vi "LlenarTabla.vi"(8 "error in (no error)":errorcluster, 11 "Prueba32 in":refnum<class "Prueba03.lvclass">) -> (0 "error out":errorcluster, 3 "Prueba32 out":refnum<class "Prueba03.lvclass">)   [LabVIEW 2019, in "Prueba03.lvclass"]
uses:
  Prueba03.lvclass
  Prueba03.lvclass/Prueba03.ctl
panel:
  out "Tabla_Ext":string[][](table)=[["63"], ["125"], ["250"], ["500"], ["1000"], ["2000"], ["4000"], ["8000"]]
  out "Tabla_Int":string[][](table)
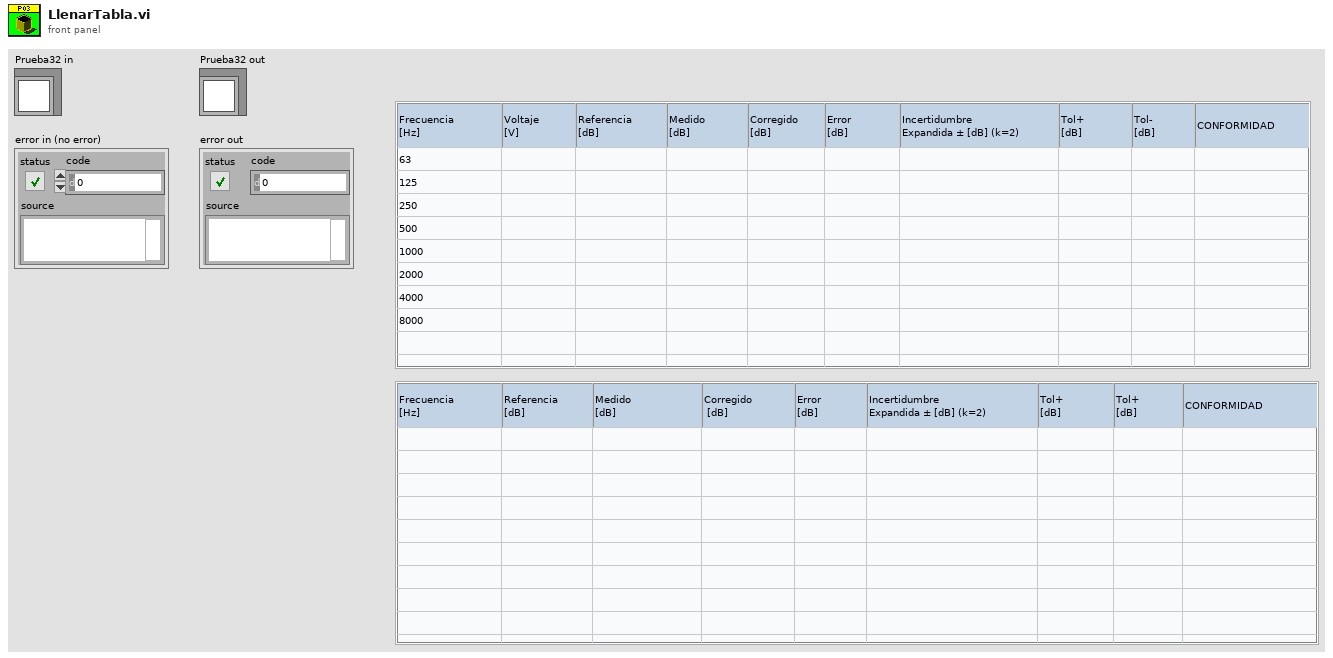
[diagram p1: front panel]
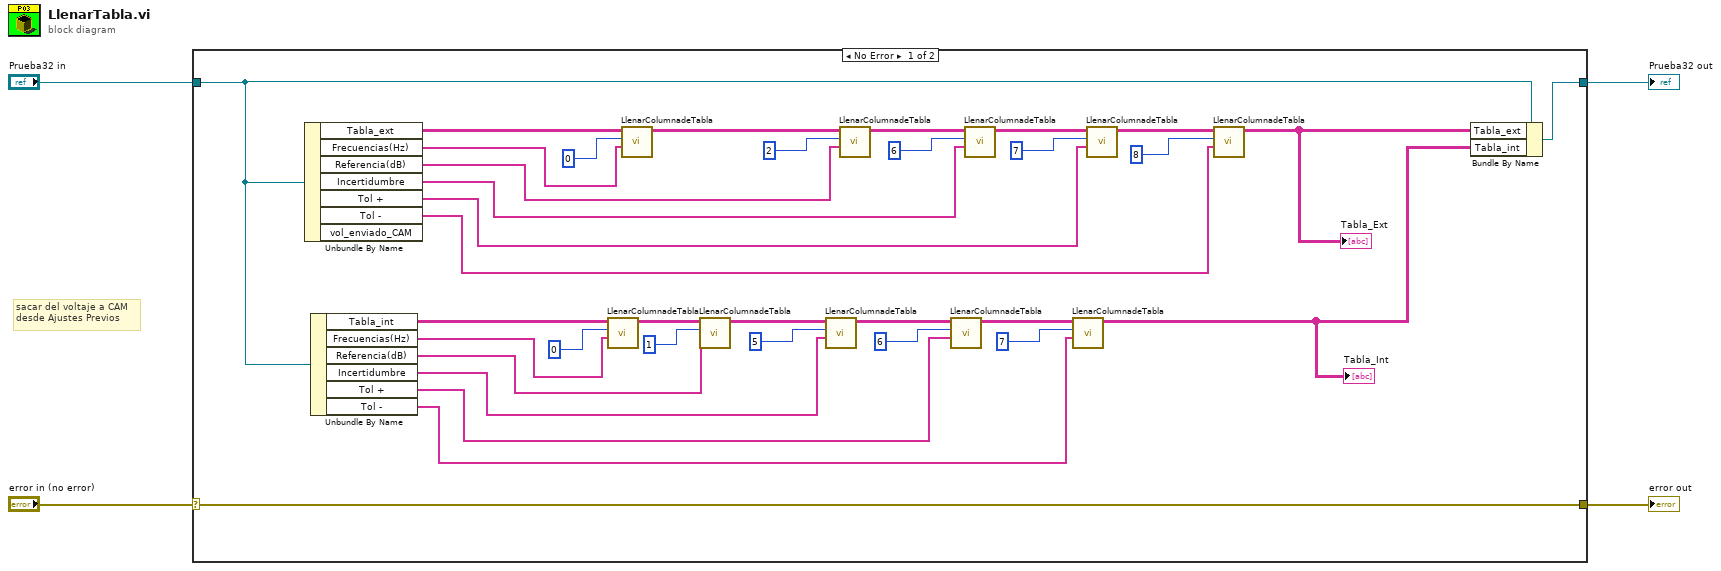
[diagram p0: block diagram]
diagram:
  # "sacar del voltaje a CAM\ndesde Ajustes Previos"
  n1 = case shown="No Error" "error in (no error)" {
    selector: "error in (no error)" -> [w39 w40]
    tunnel: [w39 w40] -> w2
    tunnel: [w37 w41] -> w3
    tunnel: "Prueba32 in" -> [w22 w41]
    frame No Error {
      n2 = Unbundle By Name(w22) -> ("Tabla_ext"=w38:string[][], "Frecuencias(Hz)"=w29:string[], "Referencia(dB)"=w23:string[], "Incertidumbre"=w28:string[], "Tol +"=w27:string[], "Tol -"=w26:string[])  [unwired: 1 out]
      n3 = Unbundle By Name(w22) -> ("Tabla_int"=w12:string[][], "Frecuencias(Hz)"=w7:string[], "Referencia(dB)"=w11:string[], "Incertidumbre"=w10:string[], "Tol +"=w9:string[], "Tol -"=w8:string[])
      n4 = call "LlenarColumnadeTabla.vi"("Data"=w7, "Col. Number"=0, "Tabla in"=w12) -> ("Tabla out"=w14:string[][])  [unwired: 8 in]
      n5 = call "LlenarColumnadeTabla.vi"("Data"=w29, "Col. Number"=0, "Tabla in"=w38) -> ("Tabla out"=w35:string[][])  [unwired: 8 in]
      n6 = call "LlenarColumnadeTabla.vi"("Data"=w11, "Col. Number"=1, "Tabla in"=w14) -> ("Tabla out"=w20:string[][])  [unwired: 8 in]
      n7 = call "LlenarColumnadeTabla.vi"("Data"=w10, "Col. Number"=5, "Tabla in"=w20) -> ("Tabla out"=w21:string[][])  [unwired: 8 in]
      n8 = call "LlenarColumnadeTabla.vi"("Data"=w23, "Col. Number"=2, "Tabla in"=w35) -> ("Tabla out"=w24:string[][])  [unwired: 8 in]
      n9 = call "LlenarColumnadeTabla.vi"("Data"=w9, "Col. Number"=6, "Tabla in"=w21) -> ("Tabla out"=w18:string[][])  [unwired: 8 in]
      n10 = call "LlenarColumnadeTabla.vi"("Data"=w28, "Col. Number"=6, "Tabla in"=w24) -> ("Tabla out"=w30:string[][])  [unwired: 8 in]
      n11 = call "LlenarColumnadeTabla.vi"("Data"=w8, "Col. Number"=7, "Tabla in"=w18) -> ("Tabla out"=w6:string[][])  [unwired: 8 in]
      "Tabla_Int" <- w6
      n12 = call "LlenarColumnadeTabla.vi"("Data"=w27, "Col. Number"=7, "Tabla in"=w30) -> ("Tabla out"=w34:string[][])  [unwired: 8 in]
      n13 = call "LlenarColumnadeTabla.vi"("Data"=w26, "Col. Number"=8, "Tabla in"=w34) -> ("Tabla out"=w5:string[][])  [unwired: 8 in]
      "Tabla_Ext" <- w5
      n14 = Bundle By Name(cluster=w22, "Tabla_ext"=w5, "Tabla_int"=w6) -> (w37:refnum<class "Prueba03.lvclass">)
    }
    frame Error {
    }
  }
  "Prueba32 out" <- w3
  "error out" <- w2
